vi "Control System - State Machine.vi"() -> ()   [LabVIEW 2021]
uses:
  <vilib>/Simulation/Scripting/Companion Diagram/SimConfigNode/SimParams.ctl
  <vilib>/Simulation/Scripting/Companion Diagram/SimConfigNode/_simSolvers.ctl
  <vilib>/Simulation/Implementation/Shared/SIMSCR Execution Mode.ctl
  <vilib>/Simulation/Param Hierarchy/Typedefs/SIMPH Param Control Actions.ctl
  <vilib>/Simulation/Implementation/Shared/NILVSim_ParamChanged.vi
  <vilib>/Simulation/Implementation/Shared/NILVSIM_BeginStep.vi
  <vilib>/Simulation/Implementation/Shared/NILVSim_Manager.vi
  <vilib>/Utility/error.llb/Clear Errors.vi
  <vilib>/Simulation/Implementation/Shared/NILVSim_FinalizeModel.vi
  <vilib>/Simulation/Implementation/Shared/SIM Unbundle Sim Info.vi
  <vilib>/Simulation/Implementation/Shared/NILVSim_Initialize.vi
  <vilib>/Simulation/Utility/Implementation/NILVSim Get Time and IsAcceptedStep.vi
  <vilib>/Simulation/Implementation/Shared/SIMSH Read Queue.vi
  <vilib>/Simulation/Implementation/Shared/NILVSim_GetModelError.vi
  <vilib>/Simulation/Implementation/Shared/SIM Bundle Sim Info.vi
  <vilib>/addons/control/pid/pid.llb/PID Advanced (DBL).vi
  <vilib>/Simulation/Implementation/XNodeFramework/SimXNode/SimX.xnode
  SubVIs/First Order Model - SubSystem.vi
  <vilib>/Simulation/Scripting/Companion Diagram/SimConfigNode/SimDog.xnode
  <vilib>/addons/control/pid/NI_PID_pid.lvlib
  <vilib>/Simulation/Implementation/Shared/NI_SIM_Implementation.lvlib
panel:
  in  "Process Parameters":cluster{"a":dbl, "b":dbl}={"a"=0.25, "b"=2.0}
  in  "PID Parameters":cluster{"Kp":dbl, "Ti [s]":dbl, "Td [s]":dbl}={"Kp"=0.1, "Ti [s]"=2.0, "Td [s]"=0.0}
  in  "Setpoint []":dbl=4.0
  in  "Stop Button":bool
  out "Waveform Chart":dbl(graph)
  out "Process Value []":dbl format="%.2g"
  out "Control Value [V]":dbl=1.0 format="%.2g"
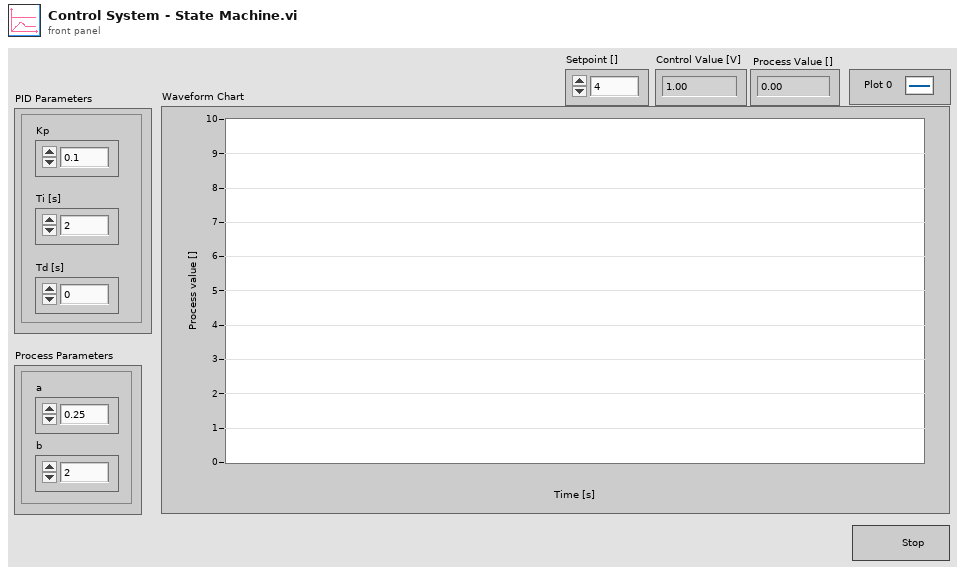
[diagram p1: front panel]
types:
  T1 = enum16{"Simulate to Completion", "Single Time-Step Simulation (Fixed Step Only)"}
  T2 = typedef "SIMSCR Execution Mode.ctl" = enum16{"Simulate to Completion", "Single Time-Step Simulation (Fixed Step Only)"}
  T3 = typedef "SIMPH Param Control Actions.ctl" = enum16{"get params", "set params"}
  T4 = cluster{"SIMSH Sim Time":dbl, "Multiplication 2":cluster{"Result":dbl}, "Multiplication":cluster{"Result":dbl}, "Summation":cluster{"Result":dbl}, "Integrator":cluster{"output":dbl}}
  T5 = typedef "SimParams.ctl" = cluster{"Initial Time (s)":dbl, "Final Time (s)":dbl, "Step Size (s)":dbl, "ODE Solver":T6, "Minimum Step Size (s)":dbl, "Maximum Step Size (s)":dbl, "Relative Tolerance":dbl, "Absolute Tolerance":dbl, "Software Timing":bool, "Initial Step Size (s)":dbl, "Automatic Fixed Step Size?":bool, "Automatic Discrete Step Size?":bool, "Discrete Step Size (s)":dbl, "Calculate using Time Step":bool, "Solver Wired?":bool, "Prev.Frm.Expected End":u64, "Prev.Frm.Actual End":u64, "Prev.Frm.Finished Late?":bool, "Prev.Iter.Expected End":u64, "Prev.Iter.Actual End":u64, "Prev.Iter.Finished Late?":bool, "Expected Iteration Start":u64, "Actual Iteration Start":u64, "Expected Frame Start":u64, "Actual Frame Start":u64, "Source Name":string, "Name":string, "Period":i64, "Deadline":i64, "Offset":i64, "Start":i64, "Priority":i32, "Timeout":i32, "Processor":i32, "Mode":enum32{"No Change", "Process missed periods, maintain original phase", "Discard missed periods, maintain original phase", "Process missed periods, ignore original phase", "Discard missed periods, ignore original phase"}, "Wakeup reason":enum32{"Normal", "Aborted", "Asynchronous wakeup", "Timing source error", "Timed loop error", "Timeout"}, "Error":errorcluster, "Source Type":string, "Secondary Source Type":string, "Global End Time":u64, "Global Start Time":u64, "Full Solver Reset":bool, "Execution Mode":T2, "Nan/Inf Check":bool, "Custom Solver Library":string, "Solver Is Variable":bool, "custom solver name":string, "Signal Collection Decimation":u32}
  T6 = typedef "_simSolvers.ctl" = enum16{"Runge-Kutta 1 (Euler)", "Runge-Kutta 2", "Runge-Kutta 3", "Runge-Kutta 4", "Runge-Kutta 23 (variable)", "Runge-Kutta 45 (variable)", "BDF (variable)", "Adams-Moulton (variable)", "Rosenbrock (variable)", "Discrete States Only", "SDIRK 4 (variable)", "Radau 5 (variable)", "Radau 9 (variable)", "Radau 13 (variable)", "Radau [Variable Order] (variable)", "Gear's Method (variable)", "Linearizer", "State Query", "Trim Eval", "Custom Solver"}
  T7 = cluster{"Kp Scaling":dbl, "Ti Scaling":dbl, "Td Scaling":dbl}
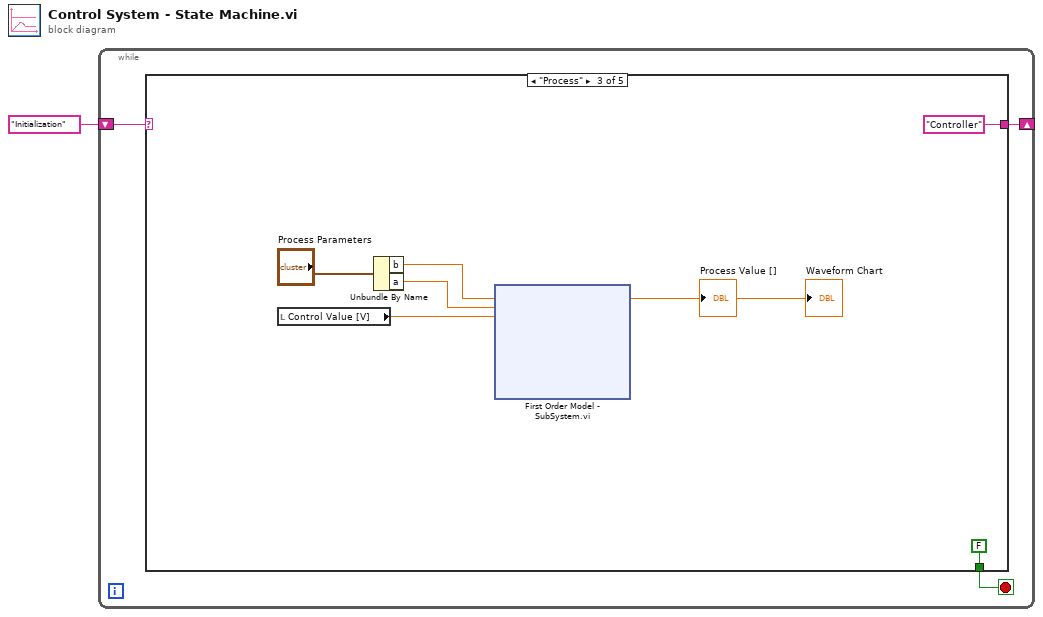
[diagram p0: block diagram]
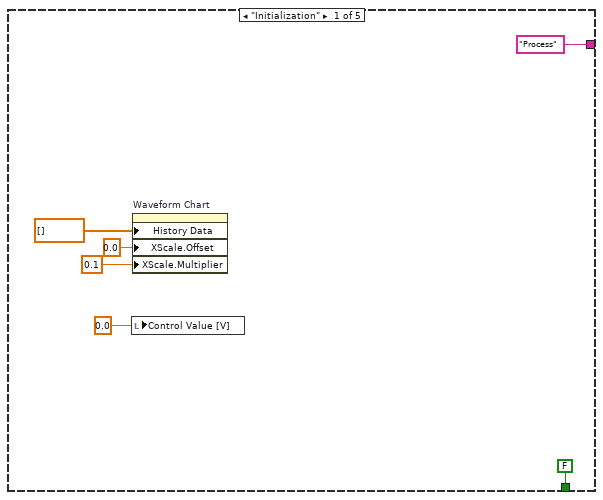
[diagram p2: hidden frame]
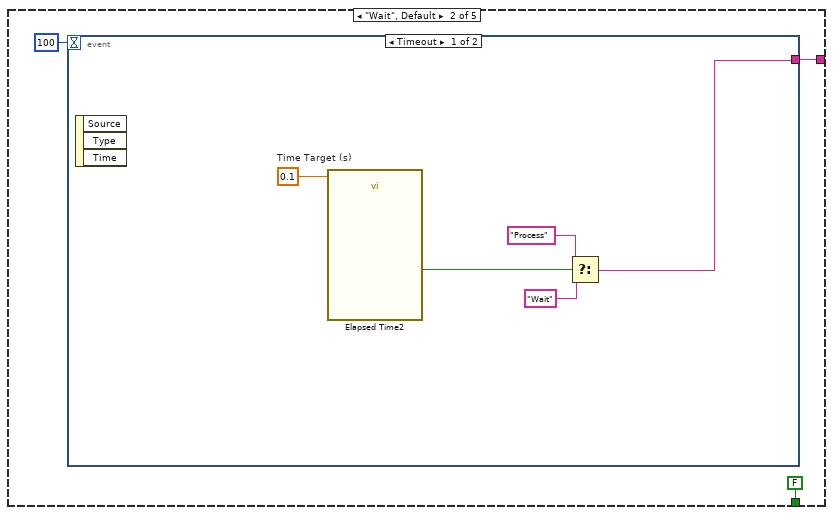
[diagram p3: hidden frame]
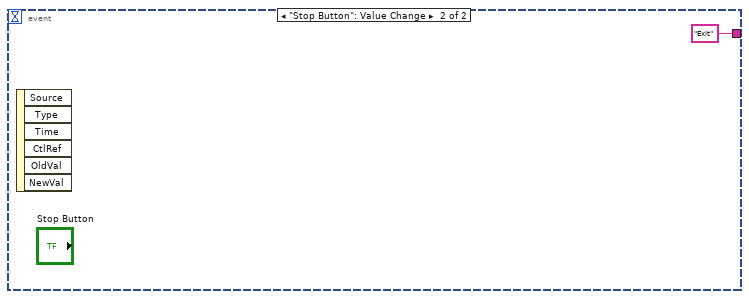
[diagram p4: hidden frame]
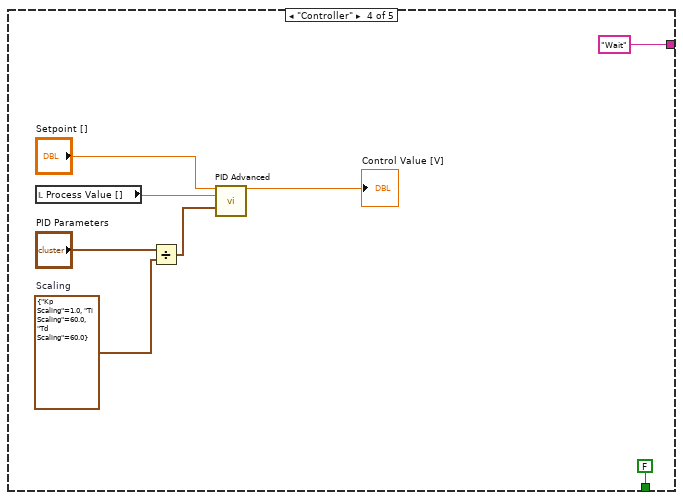
[diagram p5: hidden frame]
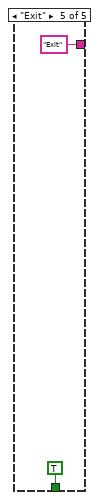
[diagram p6: hidden frame]
diagram:
  n1 = while {
    shift-right: [w3] -> _
    shift-left: "Initialization" -> [w4]
    stop <- w2 stop-if-true
    n2 = case shown="\"Process\"" w4 {
      tunnel: ["Process" w12 "Controller" "Wait" "Exit"] -> w3
      tunnel: [FALSE FALSE FALSE FALSE TRUE] -> w2
      frame "Initialization" {
        n3 = local write "Control Value [V]"(0.0 ("Control Value")) -> ()
        n4 = property on="Waveform Chart" class="WFChart (strict)"("History Data"=dbl[] [], "XScale.Offset"=0.0 ("X Scale.Offset and Multiplier:Offset"), "XScale.Multiplier"=0.1 ("X Scale.Offset and Multiplier:Multiplier")) -> ()  [unwired: 2 in, 2 out]
      }
      frame "Wait", Default {
        n5 = event shown="[0] Timeout" {
          selector: _ -> [_ _]
          dyn-events: _ -> [_ _]
          timeout: 100 -> [_ _]
          tunnel: [w14 "Exit"] -> w12
          event Timeout {
            w15 = 0.1  # Time Target (s)
            n6 = event-data() -> ()  [unwired: 1 in, 3 out]
            n7 = call "Elapsed Time2"("Time Target (s)"=w15) -> ("Time has Elapsed"=w18:bool)  [unwired: 11 in, 7 out]
            n8 = Select(t="Process", s=w18, f="Wait") -> (s? t:f=w14:string)
          }
          event "Stop Button": Value Change {
            n9 = event-data() -> ()  [unwired: 1 in, 6 out]
          }
        }
      }
      frame "Process" {
        n10 = local read "Control Value [V]"() -> (w20:dbl)
        n11 = Unbundle By Name("Process Parameters") -> ("b"=w23:dbl, "a"=w24:dbl)
        n12 = xnode "First Order Model - SubSystem.vi"("b"=w23, "a"=w24, "u"=w20) -> ("x"=→"Process Value []" →"Waveform Chart":dbl)  [unwired: 2 in, 1 out]
      }
      frame "Controller" {
        w283 = T7 {"Kp Scaling"=1.0, "Ti Scaling"=60.0, "Td Scaling"=60.0}  # Scaling
        n13 = local read "Process Value []"() -> (w281:dbl)
        n14 = Divide(x="PID Parameters", y=w283) -> (x/y=w286:cluster{dbl, dbl, dbl})
        n15 = call-poly <vilib>:"PID Advanced.vi"("setpoint"="Setpoint []", "process variable"=w281, "PID gains"=w286) -> ("output"=→"Control Value [V]":dbl)  [unwired: 11 in, 1 out]
      }
      frame "Exit" {
      }
    }
  }
